vi "test Initialize Buffer IDs.vi"(8 "error in (no error)":errorcluster) -> (0 "error out":errorcluster)   [LabVIEW 2020, in "Create Execution Unit.lvclass"]
uses:
  Create Execution Unit.lvclass
  <vilib>/addons/_JKI Toolkits/VI Tester/TestCase.llb/TestCase.lvclass
  Engine/Implementation/Rx Execution Unit/Rx Execution Unit.lvclass
  1896f177-20d1-40d1-b2fa-a279111130cc.vi
  6e7d6a2b-3dab-48ba-86cc-d2373dd18bb4.vi
  Engine/Implementation/Tx Execution Unit/Tx Execution Unit.lvclass
  Scripting/AIM MIL-STD-1553 Scripting.lvlib
  Shared/Parameter Definition.ctl
  Shared/Address.ctl
  Shared/Terminal Endpoint.ctl
  Shared/Message Type.ctl
  Shared/Message Definition.ctl
  C:/Program Files (x86)/National Instruments/LabVIEW 2020/vi.lib/addons/_JKI Toolkits/VI Tester/TestCase.llb/TestCase.lvclass
panel:
  in  "TestCase in":refnum<class "Create Execution Unit.lvclass">
  out "TestCase out":refnum<class "Create Execution Unit.lvclass">
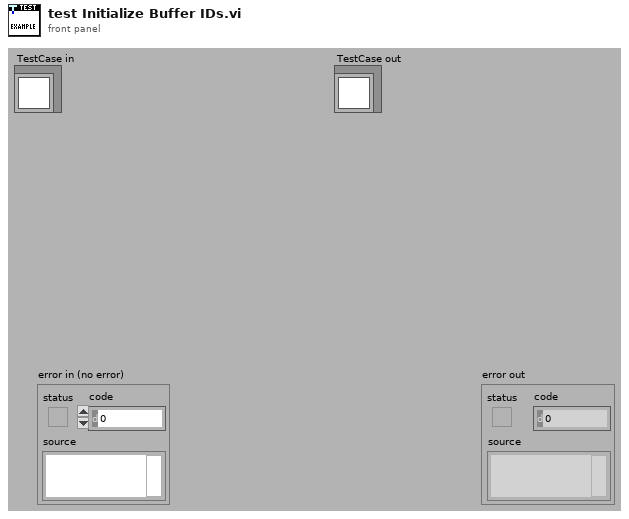
[diagram p1: front panel]
types:
  T1 = typedef "Message Definition.ctl" = cluster{"name":string, "message type":T2, "endpoint Tx":T3, "endpoint Rx":T3, "create timestamp channel":bool, "mode code":u16, "number of words":u16, "parameters":cluster{"name":string, "default value":dbl, "unit":string, "parameter definition":T5}[]}
  T2 = typedef "Message Type.ctl" = string
  T3 = typedef "Terminal Endpoint.ctl" = cluster{"terminal address":T4, "subaddress":T4}
  T4 = typedef "Address.ctl" = u16
  T5 = typedef "Parameter Definition.ctl" = cluster{"start index":i32, "size (bits)":i32, "encoding":enum16{"BNR", "BCD", "Discrete"}, "signed":bool, "multiplier":dbl, "offset":dbl}
  T6 = typedef "Custom Device API.lvlib/Custom Device Item Ref.ctl" = u64
  T7 = typedef "AIM MIL-STD-1553 Engine.lvlib/Custom Device.lvlib/Compiled Message.ctl" = cluster{"Message Section Handle":T6, "First Parameter Index":i32, "Parameter Channel Handles":T6[], "Direction":T8, "Parameters":T5[], "Receiving RT Address":u8, "Receiving RT Sub-address":u8, "Transmitting RT Address":u8, "Transmitting RT Sub-address":u8, "Word Count":u8, "Buffer Type":enum16{"unknown", "BC Message Buffer", "RT Message Buffer"}, "Buffer ID":u16, "Terminal Type":enum16{"Bus Controller", "Remote Terminal"}, "Timestamp Enabled":bool, "Timestamp Channel Handle":T6}
  T8 = typedef "Direction.ctl" = enum16{"Rx", "Tx"}
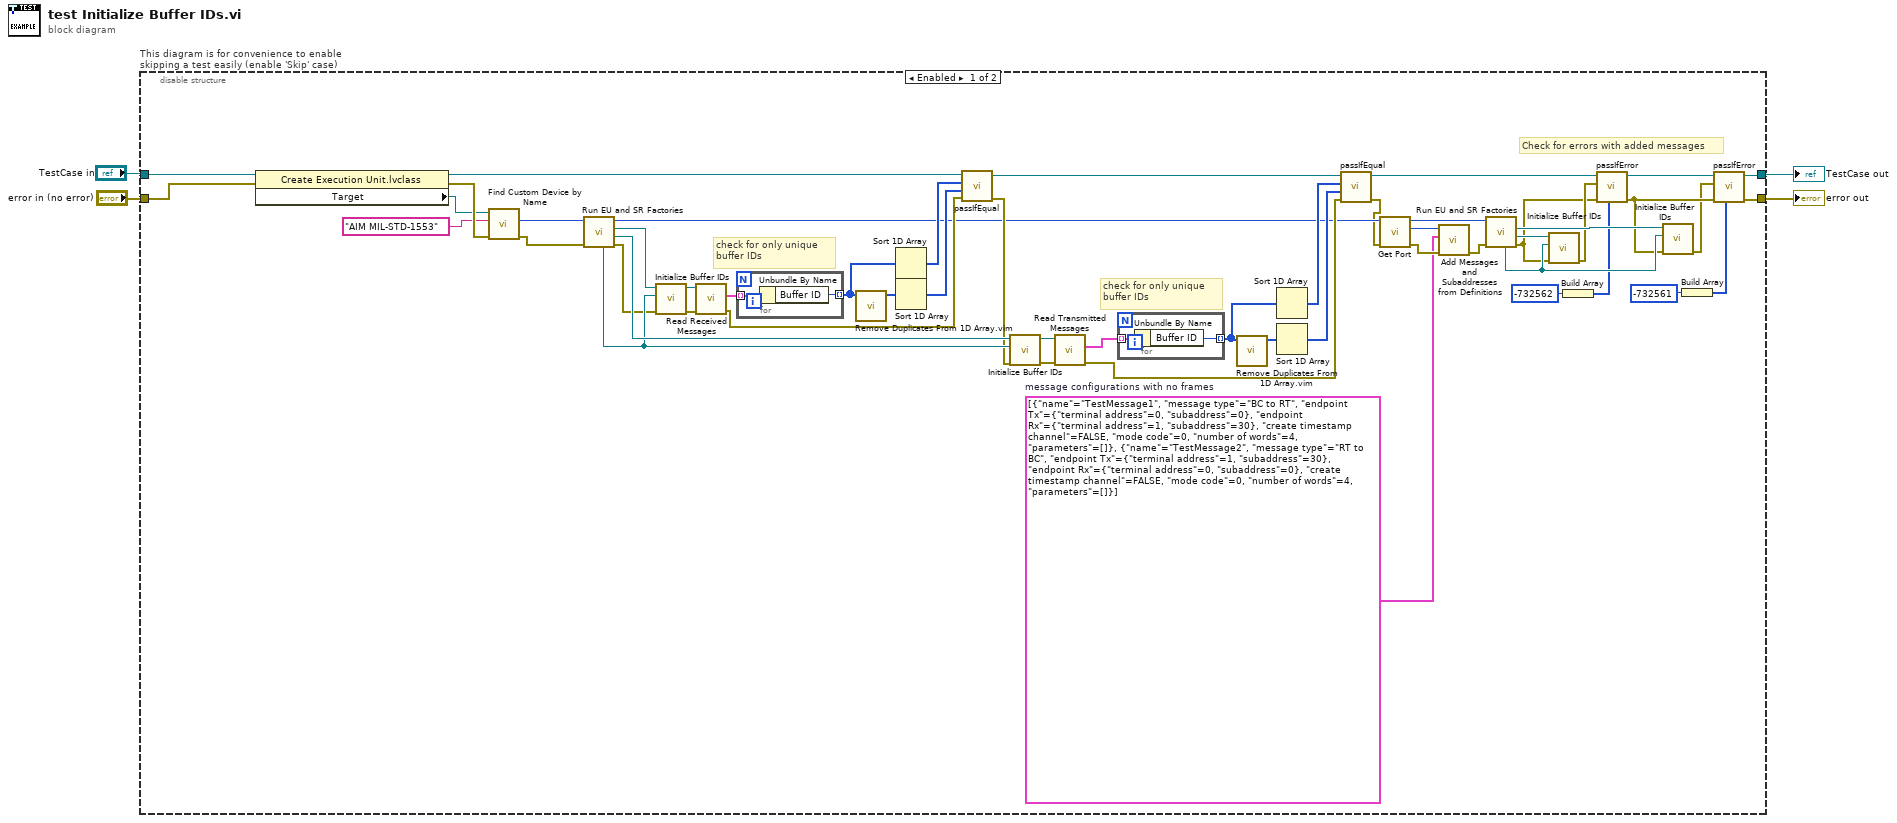
[diagram p0: block diagram]
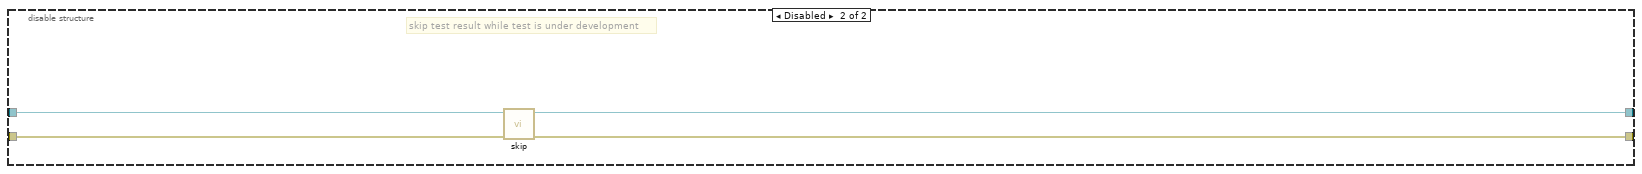
[diagram p2: hidden frame]
diagram:
  n1 = disable-structure "This diagram is for convenience to enable skipping a test easily (enable 'Skip' case)" shown="Enabled" {
    disable-tunnel: "TestCase in" -> [w52 w64]
    disable-tunnel: [w22 w62] -> w1
    disable-tunnel: [w12 w63] -> w3
    disable-tunnel: "error in (no error)" -> [w53 w61]
    frame Enabled {
      w11 = T1[] [{"name"="TestMessage1", "message type"="BC to RT", "endpoint Tx"={"terminal address"=0, "subaddress"=0}, "endpoint Rx"={"terminal address"=1, "subaddress"=30}, "create timestamp channel"=FALSE, "mode code"=0, "number of words"=4, "parameters"=[]}, {"name"="TestMessage2", "message type"="RT to BC", "endpoint Tx"={"terminal address"=1, "subaddress"=30}, "endpoint Rx"={"terminal address"=0, "subaddress"=0}, "create timestamp channel"=FALSE, "mode code"=0, "number of words"=4, "parameters"=[]}]  # message configurations with no frames
      # "Check for errors with added messages"
      # "check for only unique \nbuffer IDs"
      # "check for only unique \nbuffer IDs"
      n2 = property class="Create Execution Unit.lvclass"(reference=w52, error in=w53) -> (reference out=w51:refnum<class "Create Execution Unit.lvclass">, error out=w56:errorcluster, "Target"=w55:refnum<k24>)
      n3 = call "Find Custom Device by Name.vi"("error in"=w56, "custom device name"="AIM MIL-STD-1553" ("name"), "target"=w55) -> ("error out"=w5:errorcluster, "custom device"=w6:T6)  [unwired: 5 in, 2 out]
      n4 = call "Run EU and SR Factories.vi"("error in"=w5, "custom device"=w6) -> ("error out"=w29:errorcluster, "tx execution unit"=w32:refnum<class "Tx Execution Unit.lvclass">, "rx execution unit"=w33:refnum<class "Rx Execution Unit.lvclass">, "custom device out"=w28:T6, "shared resources"=w31:refnum<class "Shared Resources.lvclass">)  [unwired: 5 in]
      n5 = call "Initialize Buffer IDs.vi"("error in"=w29, "shared resources"=w31, "rx execution unit"=w33) -> ("error out"=w49:errorcluster, "rx execution unit out"=w50:refnum<class "Rx Execution Unit.lvclass">)  [unwired: 7 in]
      n6 = call "Read Received Messages.vi"("error in (no error)"=w49, "rx execution unit"=w50) -> ("error out"=w43:errorcluster, "received messages"=w48:T7[])  [unwired: 7 in, 1 out]
      n7 = for {
        tunnel: w48 -> [w58] mode=indexing
        tunnel: [w57] -> w46 mode=indexing
        n8 = Unbundle By Name(w58) -> ("Buffer ID"=w57:u16)
      }
      n9 = call "Remove Duplicates From 1D Array.vim"("array"=w46) -> ("array with duplicates removed"=w47:u16[])  [unwired: 10 in]
      n10 = Sort 1D Array(array=w46) -> (sorted array=w45:u16[])
      n11 = Sort 1D Array(array=w47) -> (sorted array=w44:u16[])
      n12 = call-dynamic "passIfEqual.vi"("error in (no error)"=w43, "y"=w44, "x"=w45, "TestCase in"=w51) -> ("error out"=w30:errorcluster, "TestCase out"=w34:refnum<class "Create Execution Unit.lvclass">)  [unwired: 6 in]
      n13 = call "Initialize Buffer IDs.vi"("error in"=w30, "shared resources"=w31, "tx execution unit"=w32) -> ("error out"=w38:errorcluster, "tx execution unit out"=w40:refnum<class "Tx Execution Unit.lvclass">)  [unwired: 7 in]
      n14 = call "Read Transmitted Messages.vi"("error in"=w38, "tx execution unit"=w40) -> ("error out"=w37:errorcluster, "transmitted messages"=w39:T7[])  [unwired: 7 in, 1 out]
      n15 = for {
        tunnel: w39 -> [w60] mode=indexing
        tunnel: [w59] -> w42 mode=indexing
        n16 = Unbundle By Name(w60) -> ("Buffer ID"=w59:u16)
      }
      n17 = call "Remove Duplicates From 1D Array.vim"("array"=w42) -> ("array with duplicates removed"=w41:u16[])  [unwired: 10 in]
      n18 = Sort 1D Array(array=w42) -> (sorted array=w36:u16[])
      n19 = Sort 1D Array(array=w41) -> (sorted array=w35:u16[])
      n20 = call-dynamic "passIfEqual.vi"("error in (no error)"=w37, "y"=w35, "x"=w36, "TestCase in"=w34) -> ("error out"=w26:errorcluster, "TestCase out"=w23:refnum<class "Create Execution Unit.lvclass">)  [unwired: 6 in]
      n21 = call "Get Port.vi"("error in"=w26, "custom device ref"=w28) -> ("error out"=w27:errorcluster, "port"=w24:T6, "custom device ref out"=w25:T6)  [unwired: 6 in, 1 out]
      n22 = call "Add Messages and Subaddresses from Definitions.vi"("error in"=w27, "message definitions"=w11, "port"=w24) -> ("error out"=w21:errorcluster)  [unwired: 7 in, 1 out]
      n23 = call "Run EU and SR Factories.vi"("error in"=w21, "custom device"=w25) -> ("error out"=w16:errorcluster, "tx execution unit"=w20:refnum<class "Tx Execution Unit.lvclass">, "rx execution unit"=w19:refnum<class "Rx Execution Unit.lvclass">, "shared resources"=w18:refnum<class "Shared Resources.lvclass">)  [unwired: 5 in, 1 out]
      n24 = call "Initialize Buffer IDs.vi"("error in"=w16, "shared resources"=w18, "tx execution unit"=w20) -> ("error out"=w17:errorcluster)  [unwired: 7 in, 1 out]
      n25 = Build Array(-732562 ("pass error code (0=any error code)")) -> (w9:i32[])
      n26 = call-dynamic "passIfError.vi"("passing error codes (default = any error code)"=w9, "error in (no error)"=w16, "error"=w17, "TestCase in"=w23) -> ("error out"=w14:errorcluster, "TestCase out"=w15:refnum<class "Create Execution Unit.lvclass">)  [unwired: 6 in]
      n27 = call "Initialize Buffer IDs.vi"("error in"=w14, "shared resources"=w18, "rx execution unit"=w19) -> ("error out"=w13:errorcluster)  [unwired: 7 in, 1 out]
      n28 = Build Array(-732561 ("pass error code (0=any error code)")) -> (w7:i32[])
      n29 = call-dynamic "passIfError.vi"("passing error codes (default = any error code)"=w7, "error in (no error)"=w14, "error"=w13, "TestCase in"=w15) -> ("error out"=w12:errorcluster, "TestCase out"=w22:refnum<class "Create Execution Unit.lvclass">)  [unwired: 6 in]
    }
    frame Disabled {
      # "skip test result while test is under development"
      n30 = call <vilib>:"skip.vi"("error in (no error)"=w61, "TestCase in"=w64) -> ("error out"=w63:errorcluster, "TestCase out"=w62:refnum<class "Create Execution Unit.lvclass">)  [unwired: 8 in]
    }
  }
  "error out" <- w3
  "TestCase out" <- w1
